vi "DFD Narrowband Filter Design.vi"(6 "fs [Hz]":dbl=1.0 format="%.2f", 7 "filter type":T9(ring), 8 "error in (no error)":errorcluster, 9 "ripple specs":T7={"passband"=0.05, "stopband"=60.0, "dB/linear? (T: dB)"=TRUE}, 10 "freq specs [Hz]":T8={"fpass 1"=0.015, "fstop 1"=0.02, "fpass 2 "=0.0, "fstop 2"=0.0}) -> (0 "error out":errorcluster, 3 "narrowband filter out":T1 {"multirate filters"."mMRate_SumWl" min=1 max=32 step=1; "multirate filters"."mMRate_InputIwl" min=1 max=32 step=1; "multirate filters"."mMRate_GainWl" min=1 max=32 step=1; "multirate filters"."mMRate_OutputWl" min=1 max=32 step=1; "multirate filters"."mMRate_InputWl" min=1 max=32 step=1; "multirate filters"."mMRate_CoefWl" min=1 max=32 step=1; "multirate filters"."mMRate_Mode" items=["Default"=-1, "No Rate Change"=0, "Interpolation"=1, "Decimation"=2, "Interpolated"=3, "Rational"=4]})   [LabVIEW 2017, in "NI_DigFilterLicensed.lvlib"]
doc: "Creates a narrowband filter using the interpolated finite impulse response (FIR) technique."
uses:
  <vilib>/addons/Digital Filter Design/NI_DigFilterLicensed.lvlib
  <vilib>/addons/Digital Filter Design/_Objects.llb/DFD Filter Frequence Specification (Design).ctl
  <vilib>/addons/Digital Filter Design/_Objects.llb/DFD Filter Ripple Specification (Design).ctl
  <vilib>/addons/Digital Filter Design/_Objects.llb/DFD Narrowband Filter Obj.ctl
  <vilib>/addons/Digital Filter Design/_Objects.llb/DFD Multirate Filter Obj.ctl
  <vilib>/addons/Digital Filter Design/_Objects.llb/DFD Multirate Mode.ctl
  <vilib>/addons/Digital Filter Design/_Objects.llb/DFD Coef Norm Type.ctl
  <vilib>/addons/Digital Filter Design/_Objects.llb/DFD Round-off Mode.ctl
  <vilib>/addons/Digital Filter Design/_Objects.llb/DFD FXP MRate Multiply Mode.ctl
  <vilib>/addons/Digital Filter Design/NI_DigFilter_Process.lvlib
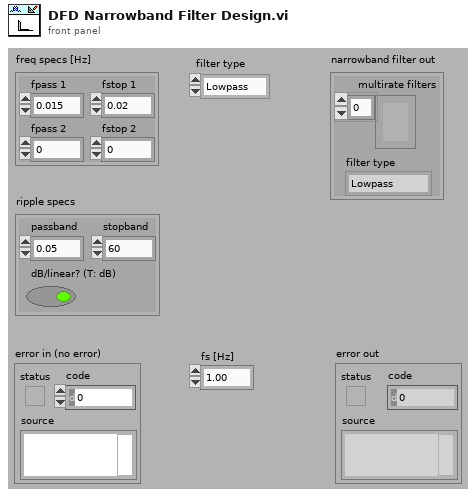
[diagram p1: front panel]
types:
  T1 = typedef "NI_DigFilterLicensed.lvlib/DFD Narrowband Filter Obj.ctl" = cluster{"multirate filters":T2[], "filter type":enum32{"Lowpass", "Highpass", "Bandpass", "Bandstop", "Wideband-Lowpass", "Wideband-Highpass"}}
  T2 = typedef "NI_DigFilterLicensed.lvlib/DFD Multirate Filter Obj.ctl" = cluster{"mMRate_Structure":enum16{"CIC", "FIR", "IIR", "Lattice"}, "mMRate_Mode":T3, "mMRate_Factor":i32, "mMRate_FIRParams":cluster{"mMRate_FIR_H":dbl[], "mMRate_FIR_IsNyquist?":bool, "mMRate_FIR_IsSymmetric?":bool}, "mMRate_CICParams":cluster{"mMRate_CIC_#Stage":i32, "mMRate_CIC_Lag":i32, "mMRate_CIC_Type":enum16{"Lowpass", "Highpass"}}, "mMRate_Order":i32, "mMRate_Version":string, "mMRate_Comments":string, "mMRate_RationalFactor":cluster{"mMRate_L":i32, "mMRate_M":i32}, "mMRate_Fs":dbl, "mMRate_Quantized?":bool, "mMRate_QFilterGain":dbl, "mMRate_CoefWl":i16, "mMRate_Scaling":cluster{"mMRate_ScaleByPowerOf2?":bool, "mMRate_ScaleType":T4}, "mMRate_InputWl":i16, "mMRate_OutputWl":i16, "mMRate_OutputMode":T5, "mMRate_MultMode":T6, "mMRate_BitPruning":bool, "mMRate_GainWl":i16, "mMRate_OutputFwl":i16, "mMRate_SumIwl":i16, "mMRate_InputIwl ":i16, "mMRate_SumWl":i16, "mMRate_CoefIwl":i16}
  T3 = typedef "NI_DigFilterLicensed.lvlib/DFD Multirate Mode.ctl" = i16
  T4 = typedef "NI_DigFilterLicensed.lvlib/DFD Coef Norm Type.ctl" = enum16{"No Norm", "Time Domain 1-Norm", "Time Domain 2-Norm", "Time Domain Inf-Norm"}
  T5 = typedef "NI_DigFilterLicensed.lvlib/DFD Round-off Mode.ctl" = enum16{"Nearest", "Truncation"}
  T6 = typedef "NI_DigFilterLicensed.lvlib/DFD FXP MRate Multiply Mode.ctl" = enum16{"Truncated", "Full"}
  T7 = typedef "NI_DigFilterLicensed.lvlib/DFD Filter Ripple Specification (Design).ctl" = cluster{"passband":dbl, "stopband":dbl, "dB/linear? (T: dB)":bool}
  T8 = typedef "NI_DigFilterLicensed.lvlib/DFD Filter Frequence Specification (Design).ctl" = cluster{"fpass 1":dbl, "fstop 1":dbl, "fpass 2 ":dbl, "fstop 2":dbl}
  T9 = enum16{"Lowpass", "Highpass", "Bandpass", "Bandstop"}
  T10 = enum32{"Lowpass", "Highpass", "Bandpass", "Bandstop", "Wideband-Lowpass", "Wideband-Highpass"}
  T11 = cluster{"multirate filter out":T2[], "new filter type":enum32{"Lowpass", "Highpass", "Bandpass", "Bandstop", "Wideband-Lowpass", "Wideband-Highpass"}}
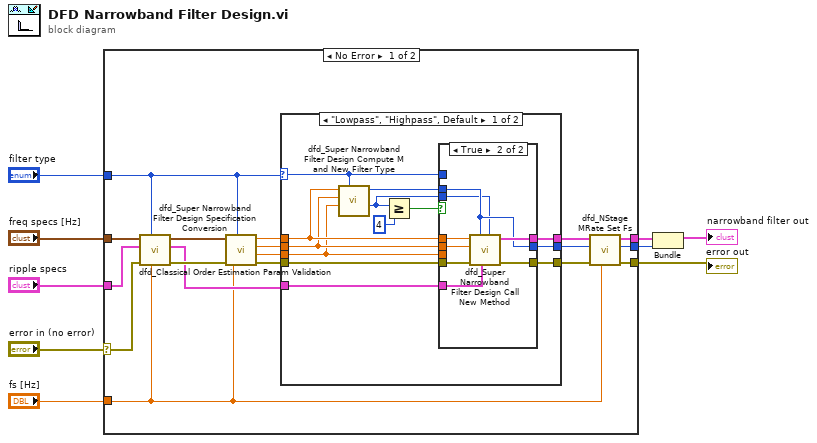
[diagram p0: block diagram]
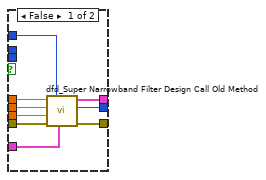
[diagram p2: hidden frame]
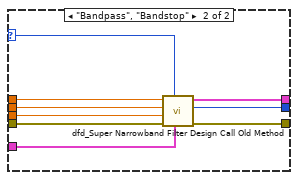
[diagram p3: hidden frame]
diagram:
  n1 = case shown="No Error" "error in (no error)" {
    selector: "error in (no error)" -> [w24 w66]
    tunnel: "filter type" -> [w26 _]
    tunnel: "freq specs [Hz]" -> [w25 _]
    tunnel: "ripple specs" -> [w15 _]
    tunnel: "fs [Hz]" -> [w11 _]
    tunnel: [w13 _] -> w1
    tunnel: [w10 w66] -> w4
    tunnel: [w17 _] -> w3
    frame No Error {
      n2 = call <vilib>:"dfd_Classical Order Estimation Param Validation.vi"("fs [Hz]"=w11, "filter type"=w26, "error in (no error)"=w24, "ripple specs"=w15, "freq specs [Hz]"=w25) -> ("error out"=w20:errorcluster, "dup ripple specs"=w14:T7, "dup freq specs [Hz]"=w16:T8)  [unwired: 4 out]
      n3 = call <vilib>:"dfd_Super Narrowband Filter Design Specification Conversion.vi"("fs [Hz]"=w11, "filter type"=w26, "error in (no error)"=w20, "freq specs [Hz]"=w16) -> ("error out"=w19:errorcluster, "fc"=w18:dbl, "fstop"=w21:dbl, "fpass"=w22:dbl)  [unwired: 1 in, 3 out]
      n4 = case shown="\"Lowpass\", \"Highpass\", Default" w26 {
        selector: w26 -> [w36 w57]
        tunnel: w19 -> [w29 w62]
        tunnel: [w39 w60] -> w12
        tunnel: [w38 w61] -> w23
        tunnel: w22 -> [w32 w65]
        tunnel: w21 -> [w31 w64]
        tunnel: w18 -> [w30 w63]
        tunnel: [w37 w59] -> w17
        tunnel: w14 -> [w28 w58]
        frame "Lowpass", "Highpass", Default {
          n5 = call <vilib>:"dfd_Super Narrowband Filter Design Compute M and New Filter Type.vi"("filter type"=w36, "fc"=w30, "fstop"=w31, "fpass"=w32) -> ("M"=w27:i32, "new filter type"=w33:T10)  [unwired: 1 in, 5 out]
          n6 = Greater Or Equal?(x=w27, y=4) -> (x >= y?=w34:bool)
          n7 = case shown="True" w34 {
            tunnel: [w48 w56] -> w38
            tunnel: [w47 w55] -> w39
            tunnel: [w46 w50] -> w37
            tunnel: w36 -> [w41 _]
            tunnel: w33 -> [_ w50]
            tunnel: w32 -> [w45 w52]
            tunnel: w31 -> [w44 w51]
            tunnel: w30 -> [w43 _]
            tunnel: w29 -> [w42 w53]
            tunnel: w28 -> [w40 w54]
            tunnel: w27 -> [_ w49]
            frame False {
              n8 = call <vilib>:"dfd_Super Narrowband Filter Design Call Old Method.vi"("ripple specs"=w40, "filter type"=w41, "error in (no error)"=w42, "fc"=w43, "fstop"=w44, "fpass"=w45) -> ("error out"=w47:errorcluster, "new filter type"=w46:T10, "multirate filters out"=w48:T2[])  [unwired: 1 in, 2 out]
            }
            frame True {
              n9 = call <vilib>:"dfd_Super Narrowband Filter Design Call New Method.vi"("M"=w49, "ripple specs"=w54, "new filter type"=w50, "error in (no error)"=w53, "fstop"=w51, "fpass"=w52) -> ("error out"=w55:errorcluster, "multirate filters out"=w56:T2[])  [unwired: 1 in, 3 out]
            }
          }
        }
        frame "Bandpass", "Bandstop" {
          n10 = call <vilib>:"dfd_Super Narrowband Filter Design Call Old Method.vi"("ripple specs"=w58, "filter type"=w57, "error in (no error)"=w62, "fc"=w63, "fstop"=w64, "fpass"=w65) -> ("error out"=w60:errorcluster, "new filter type"=w59:T10, "multirate filters out"=w61:T2[])  [unwired: 1 in, 2 out]
        }
      }
      n11 = call <vilib>:"dfd_NStage MRate Set Fs.vi"("fs in [Hz]"=w11, "error in (no error)"=w12, "multirate filter in"=w23) -> ("error out"=w10:errorcluster, "multirate filter out"=w13:T2[])  [unwired: 7 out]
    }
    frame Error {
    }
  }
  "error out" <- w4
  n12 = Bundle("multirate filter out"=w1, "new filter type"=w3) -> (→"narrowband filter out":T11)  [unwired: 1 out]
